vi "XY Graph Find Plot Zero-Crossing Location.vi"(8 "Error In":errorcluster, 10 "Y Array":dbl[](array[numeric]), 11 "X Array":dbl[](array[numeric])) -> (0 "Error Out":errorcluster, 1 "Location Index":dbl, 3 "Zero Crossing Location":dbl)   [LabVIEW 2021, in "XY Graph Add-Ons.lvlib"]
uses:
  <vilib>/Utility/error.llb/Error Cluster From Error Code.vi
  <vilib>/ErrorRing/Error Ring.xnode
  XY Graph Add-Ons.lvlib
panel:
  # "This handles both up-down and down-up types of crossing"
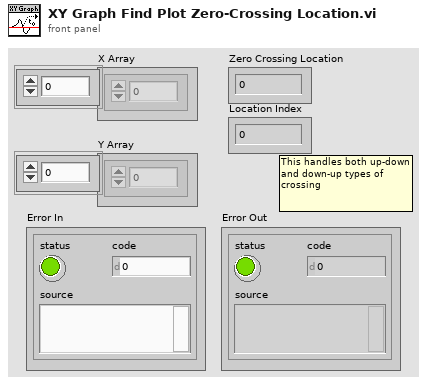
[diagram p1: front panel]
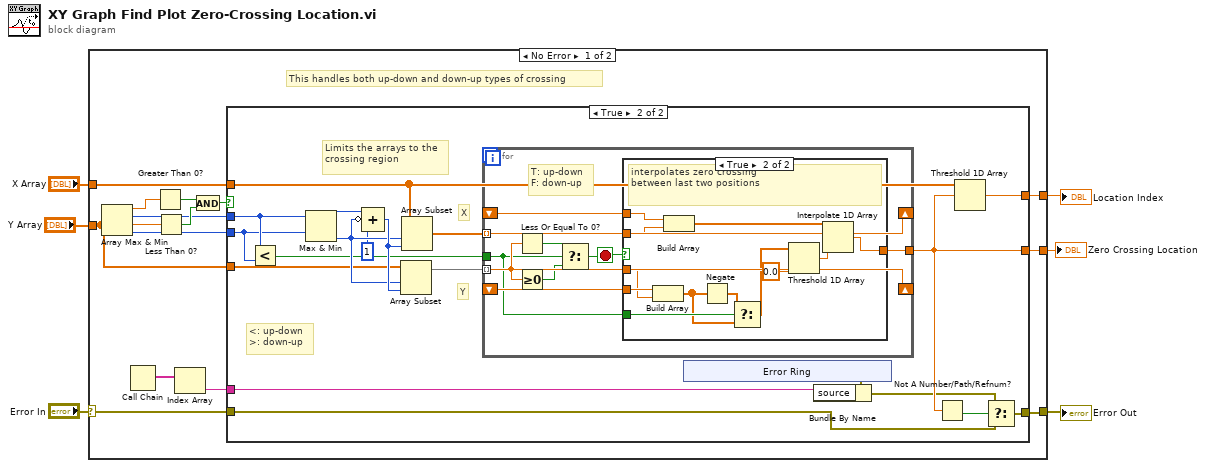
[diagram p0: block diagram]
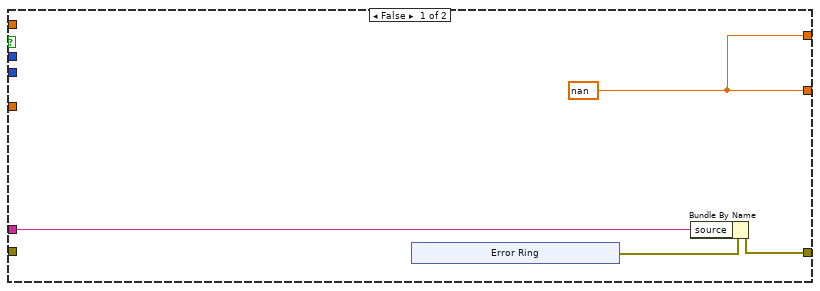
[diagram p2: hidden frame]
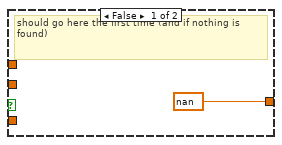
[diagram p3: hidden frame]
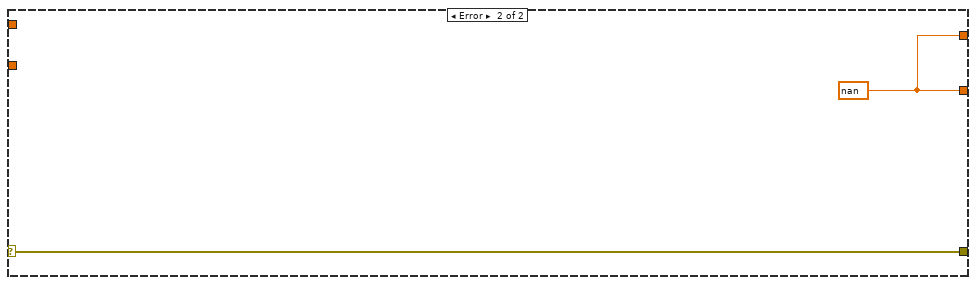
[diagram p4: hidden frame]
diagram:
  n1 = case shown="No Error" "Error In" {
    selector: "Error In" -> [w10 w75]
    tunnel: "X Array" -> [w21 _]
    tunnel: "Y Array" -> [w20 _]
    tunnel: [w19 w76] -> w4
    tunnel: [w11 w76] -> w2
    tunnel: [w9 w75] -> w1
    frame No Error {
      # "This handles both up-down and down-up types of crossing"
      n2 = Array Max & Min(array=w20) -> (max value=w15:dbl, max index (indices)=w13:i32, min value=w16:dbl, min index (indices)=w14:i32)
      n3 = Call Chain() -> (call chain=w8:string[])
      n4 = Greater Than 0?(x=w15) -> (x > 0?=w17:bool)
      n5 = Less Than 0?(x=w16) -> (x < 0?=w18:bool)
      n6 = Index Array(array=w8) -> (element=w7:string)  [unwired: 1 in]
      n7 = And(x=w17, y=w18) -> (x .and. y?=w12:bool)
      n8 = case shown="True" w12 {
        tunnel: w21 -> [_ w38]
        tunnel: w20 -> [_ w42]
        tunnel: [w25 w36] -> w19
        tunnel: w14 -> [_ w40]
        tunnel: w13 -> [_ w41]
        tunnel: [w25 w37] -> w11
        tunnel: w10 -> [_ w31]
        tunnel: [w23 w30] -> w9
        tunnel: w7 -> [w22 w34]
        frame False {
          w25 = nan
          n9 = xnode "Error Ring"() -> ("error out"=w24:errorcluster)
          n10 = Bundle By Name(cluster=w24, "source"=w22) -> (w23:errorcluster)
        }
        frame True {
          # "Y"
          # "X"
          # "<: up-down\n>: down-up"
          # "Limits the arrays to the crossing region"
          n11 = Less?(x=w41, y=w40) -> (x < y?=w39:bool)
          n12 = Max & Min(x=w41, y=w40) -> (max(x,y)=w43:i32, min(x,y)=w46:i32)
          n13 = Compound Arithmetic op=ADD(w43, invert w46, 1 ("value")) -> (w47:i32)
          n14 = Array Subset(array=w42, index=w46, length=w47) -> (w45:dbl[])
          n15 = Array Subset(array=w38, index=w46, length=w47) -> (w48:dbl[])
          n16 = for {
            tunnel: w45 -> [w55] mode=indexing
            tunnel: w48 -> [w59] mode=indexing
            shift-right: [w59] -> _
            shift-left: _ -> [w60]
            shift-right: [w55] -> _
            shift-left: _ -> [w58]
            tunnel: [w61] -> w36
            tunnel: w39 -> [w53]
            stop <- w56 stop-if-true
            # "T: up-down\nF: down-up"
            n17 = Less Or Equal To 0?(x=w55) -> (x <= 0?=w57:bool)
            n18 = Greater Or Equal To 0?(x=w55) -> (x >= 0?=w54:bool)
            n19 = Select(t=w57, s=w53, f=w54) -> (s? t:f=w56:bool)
            n20 = case shown="True" w56 {
              tunnel: [nan w67] -> w61
              tunnel: w60 -> [_ w74]
              tunnel: w59 -> [_ w73]
              tunnel: w55 -> [_ w71]
              tunnel: w58 -> [_ w72]
              tunnel: w53 -> [_ w66]
              frame False {
                # "should go here the first time (and if nothing is found)"
              }
              frame True {
                # "interpolates zero crossing\nbetween last two positions"
                n21 = Build Array(w72, w71) -> (w63:dbl[])
                n22 = Build Array(w74, w73) -> (w69:dbl[])
                n23 = Negate(x=w63) -> (-x=w65:dbl[])
                n24 = Select(t=w65, s=w66, f=w63) -> (s? t:f=w64:dbl[])
                n25 = Threshold 1D Array(2:0.0 ("threshold y"), 3:w64) -> (0:w68:dbl)  [unwired: 1 in]
                n26 = Interpolate 1D Array(1:w68, 2:w69) -> (0:w67:dbl)
              }
            }
          }
          n27 = xnode "Error Ring"() -> ("error out"=w35:errorcluster)
          n28 = Bundle By Name(cluster=w35, "source"=w34) -> (w32:errorcluster)
          n29 = Not A Number/Path/Refnum?(number/path/refnum=w36) -> (NaN/Path/Refnum?=w33:bool)
          n30 = Threshold 1D Array(2:w36, 3:w38) -> (0:w37:dbl)  [unwired: 1 in]
          n31 = Select(t=w32, s=w33, f=w31) -> (s? t:f=w30:errorcluster)
        }
      }
    }
    frame Error {
      w76 = nan
    }
  }
  "Zero Crossing Location" <- w4
  "Error Out" <- w1
  "Location Index" <- w2
